vi "DriveGetMaxSpeed_M.vi"() -> (3 "Max Speed (m/sec)":dbl)   [LabVIEW 2023]
doc: "Constant variable for max speed of robot to use in calculations"
uses:
  <vilib>/Rock Robotics/WPI/ThirdParty/JAS_Junk/TrajLib/Trajectory_Library.lvlib
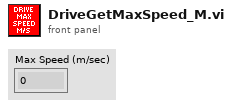
[diagram p1: front panel]
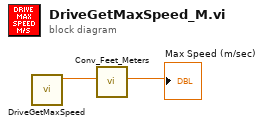
[diagram p0: block diagram]
diagram:
  n1 = call "DriveGetMaxSpeed.vi"() -> ("Max Speed (ft/sec)"=w2:dbl)  [unwired: 11 in]
  n2 = call <vilib>:"Conv_Feet_Meters.vi"("Feet"=w2) -> ("Meters"=→"Max Speed (m/sec)":dbl)  [unwired: 10 in]
